vi "I2C Grove 8x8Matrix LED.vi"() -> ()   [LabVIEW 2020, in "CTI-Scratchpad.lvlib"]
uses:
  CTI-Scratchpad.lvlib
  CTI/Identity.ctl
  CTI-Peripheral/I2CLEDMatrix/Base/Data Types/ICONS.ctl
  CTI/Error Reporting.ctl
  CTI/I2C Address.ctl
  CTI/GPIO Number.ctl
  CTI/I2C Number.ctl
  CTI/Session/Session.lvclass
  CTI-Peripheral/I2CLEDMatrix/Grove I2C 8x8LEDMatrix/Grove I2C Matrix LED Driver.lvclass
  CTI/VisaComms/VisaComms.lvclass
  CTI/CTI.lvlib
  CTI-Peripheral/I2CLEDMatrix/Base/LEDMatrix.lvclass
panel:
  out "Shifting ASCII":bool[][](array[boolean])
  in  "Char":bool[][](array[boolean])=[[FALSE, FALSE, FALSE, FALSE, FALSE], [FALSE, FALSE, FALSE, FALSE, FALSE], [FALSE, FALSE, FALSE, FALSE, FALSE], [FALSE, FALSE, FALSE, FALSE, FALSE], [FALSE, FALSE, FALSE, FALSE, FALSE], [FALSE, FALSE, FALSE, FALSE, FALSE], [FALSE, FALSE, FALSE, FALSE, FALSE], [FALSE, FALSE, FALSE, FALSE, FALSE]]
  in  "Set Custom Char":bool
  in  "Set Scrolling Text":bool
  in  "Scrolling Text":string="test"
  in  "Icon":T1
  in  "Set Icon":bool
  in  "String":string
  in  "Set Char":bool
  out "Identity":T2
  in  "stop":bool
  in  "Grove Connector":enum16{"I2C0", "I2C1"}(ring)
  out "error out":errorcluster
  in  "Port":refnum<visa-resource-name>="COM4"
  # "https://wiki.seeedstudio.com/Grove-LED_Matrix_Driver-HT16K33/"
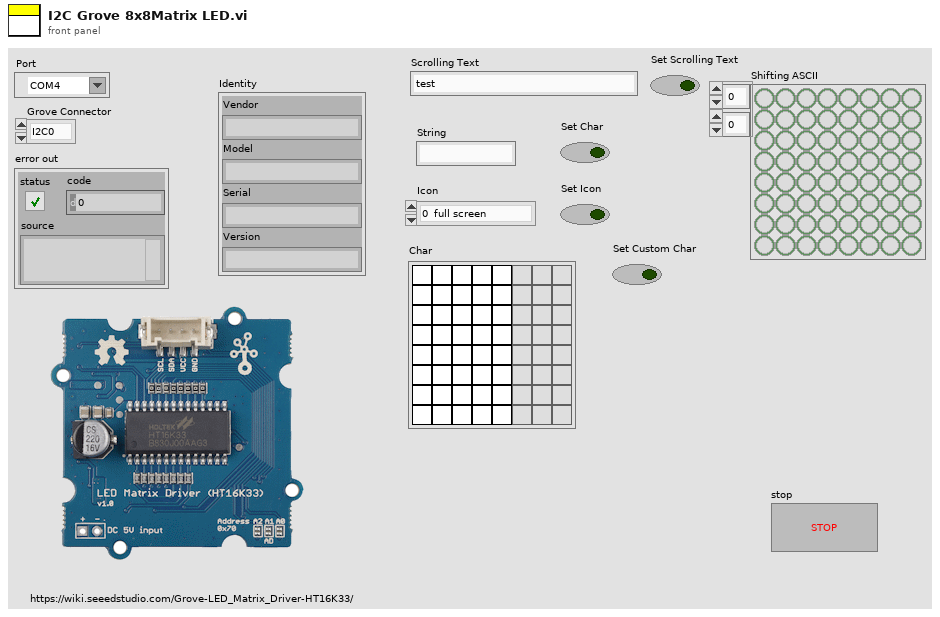
[diagram p1: front panel]
types:
  T1 = typedef "CTI-Peripheral.lvlib/LEDMatrix.lvclass/ICONS.ctl" = enum16{"0  full screen", "1  arrow_up", "2  arrow_down", "3  arrow_right", "4  arrow_left", "5  triangle_up", "6  triangle_down", "7  triangle_right", "8  triangel_left", "9  smile_face_1", "10 smile_face_2", "11 hearts", "12 diamonds", "13 clubs", "14 spades", "15 circle1", "16 circle2", "17 circle3", "18 circle4", "19 man", "20 woman", "21 musical_note_1", "22 musical_note_2", "23 snow", "24 up_down", "25 double_!", "26 left_right", "27 house"}
  T2 = typedef "CTI.lvlib/Identity.ctl" = cluster{"Vendor":string, "Model":string, "Serial":string, "Version":string}
  T3 = typedef "CTI.lvlib/I2C Address.ctl" = u8
  T4 = typedef "CTI.lvlib/Error Reporting.ctl" = enum16{"Minimal", "Moderate", "Full"}
  T5 = typedef "CTI.lvlib/I2C Number.ctl" = i8
  T6 = typedef "CTI.lvlib/GPIO Number.ctl" = i8
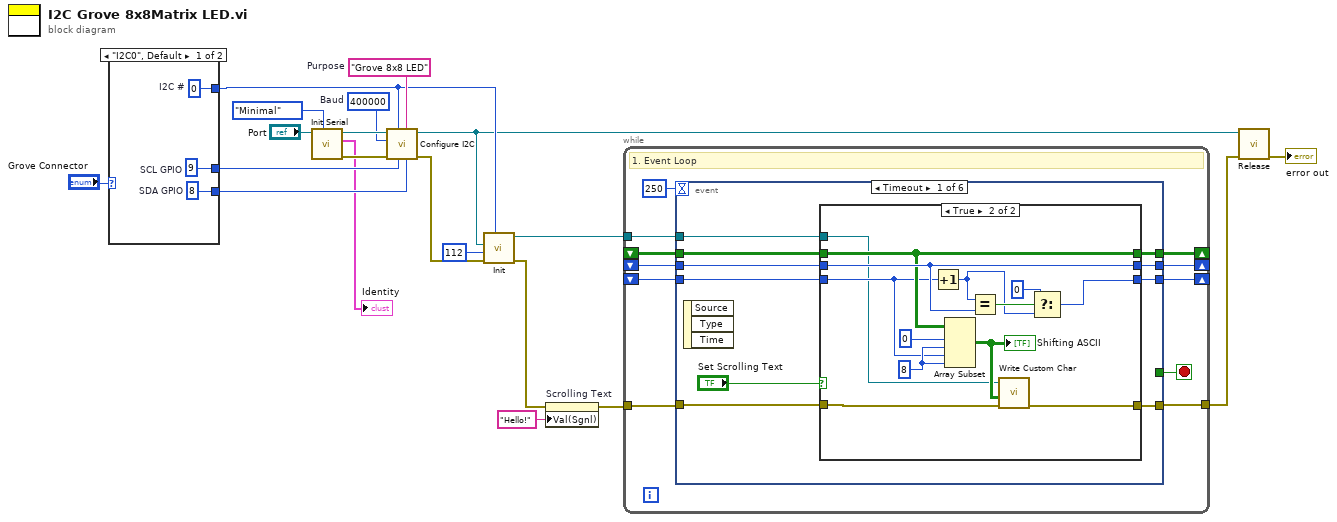
[diagram p0: block diagram]
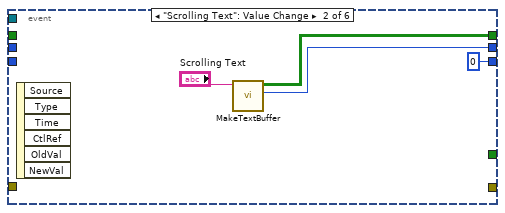
[diagram p3: hidden frame]
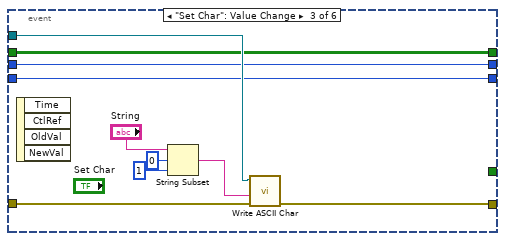
[diagram p4: hidden frame]
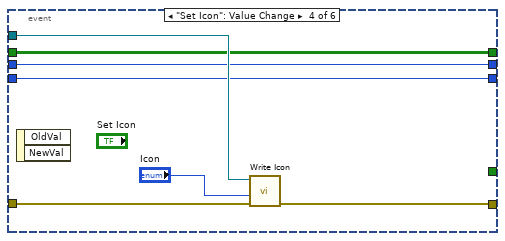
[diagram p5: hidden frame]
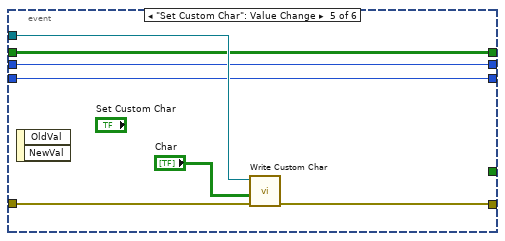
[diagram p6: hidden frame]
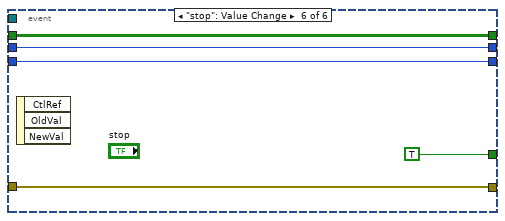
[diagram p7: hidden frame]
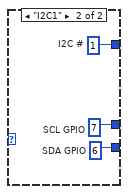
[diagram p8: hidden frame]
diagram:
  w15 = "Grove 8x8 LED"  # Purpose
  w16 = u32 400000  # Baud
  n1 = case shown="\"I2C0\", Default" "Grove Connector" {
    tunnel: [w23 w26] -> w13
    tunnel: [w22 w25] -> w12
    tunnel: [w21 w24] -> w8
    frame "I2C0", Default {
      w21 = T5 0  # I2C #
      w22 = T6 8  # SDA GPIO
      w23 = T6 9  # SCL GPIO
    }
    frame "I2C1" {
      w24 = T5 1  # I2C #
      w25 = T6 6  # SDA GPIO
      w26 = T6 7  # SCL GPIO
    }
  }
  n2 = call "Init Serial.vi"("Error Checking (Full)"=Error_Reporting."Minimal", "VISA resource name in"="Port") -> ("error out"=w17:errorcluster, "Identity"=→"Identity":T2, "Session"=w18:refnum<class "Session.lvclass">)  [unwired: 7 in]
  n3 = call "Configure I2C.vi"("SDA GPIO"=w12, "Purpose (\"I2C\")"=w15, "SCL GPIO"=w13, "I2C #"=w8, "error in (no error)"=w17, "Baud"=w16, "Session in"=w18) -> ("error out"=w5:errorcluster, "Session out"=w7:refnum<class "Session.lvclass">)  [unwired: 3 in]
  n4 = call "Init.vi"("I2C #"=w8, "error in (no error)"=w5, "Address"=T3 112, "Session In"=w7) -> ("error out"=w3:errorcluster, "Grove I2C Matrix LED Driver Out"=w4:refnum<class "Grove I2C Matrix LED Driver.lvclass">)  [unwired: 6 in]
  n5 = property on="Scrolling Text" class="Str"(error in=w3, "Val(Sgnl)"="Hello!" ("Value (Signaling)")) -> (error out=w2:errorcluster)  [unwired: 1 in, 1 out]
  n6 = while {
    tunnel: w2 -> [w36]
    tunnel: [w35] -> w10
    tunnel: w4 -> [w37]
    shift-right: [w32] -> _
    shift-left: _ -> [w31]
    shift-right: [w30] -> _
    shift-left: _ -> [w29]
    shift-right: [w27] -> _
    shift-left: _ -> [w28]
    stop <- w34 stop-if-true
    # "1. Event Loop"
    n7 = event shown="[0] Timeout" {
      selector: _ -> [_ _ _ _ _ _]
      dyn-events: _ -> [_ _ _ _ _ _]
      timeout: 250 -> [_ _ _ _ _ _]
      tunnel: w37 -> [w41 _ w76 w82 w90 _]
      tunnel: w36 -> [w40 _ w78 w85 w92 w97]
      tunnel: [w39 _ w77 w84 w91 w97] -> w35
      tunnel: [_ _ _ _ _ TRUE] -> w34
      tunnel: [w43 w67 w69 w81 w86 w93] -> w32
      tunnel: w31 -> [w44 _ w69 w81 w86 w93]
      tunnel: [w42 w66 w70 w79 w87 w94] -> w30
      tunnel: w29 -> [w45 _ w70 w79 w87 w94]
      tunnel: w28 -> [w47 _ w71 w80 w88 w95]
      tunnel: [w46 0 ("index") w71 w80 w88 w95] -> w27
      event Timeout {
        n8 = event-data() -> ()  [unwired: 1 in, 3 out]
        n9 = case shown="True" "Set Scrolling Text" {
          tunnel: w47 -> [w48 w56]
          tunnel: [w48 w62] -> w46
          tunnel: w45 -> [w49 w60]
          tunnel: w44 -> [w50 w57]
          tunnel: [w50 w57] -> w43
          tunnel: [w49 w60] -> w42
          tunnel: w41 -> [_ w52]
          tunnel: w40 -> [w51 w55]
          tunnel: [w51 w53] -> w39
          frame False {
          }
          frame True {
            w58 = 8 ("length")
            n10 = Increment(x=w56) -> (x+1=w61:i32)
            n11 = Array Subset(array=w57, index (row)=0 ("index"), length (row)=w58, index (col)=w56, length (col)=w58) -> (w54:bool[][])
            "Shifting ASCII" <- w54
            n12 = Equal?(x=w61, y=w60) -> (x = y?=w63:bool)
            n13 = call-dynamic "Write Custom Char.vi"("error in (no error)"=w55, "Char"=w54, "Grove I2C Matrix LED in"=w52) -> ("error out"=w53:errorcluster)  [unwired: 7 in, 1 out]
            n14 = Select(t=0 ("index"), s=w63, f=w61) -> (s? t:f=w62:i32)
          }
        }
      }
      event "Scrolling Text": Value Change {
        n15 = event-data() -> ()  [unwired: 1 in, 6 out]
        n16 = call "MakeTextBuffer.vi"("Text"="Scrolling Text") -> ("size"=w66:i32, "Buffer"=w67:bool[][])  [unwired: 9 in]
      }
      event "Set Char": Value Change {
        n17 = event-data() -> ()  [unwired: 1 in, 4 out]
        n18 = String Subset(string="String", offset (0)=0, length (rest)=1 ("length (rest)")) -> (substring=w72:string)
        n19 = call-dynamic "Write ASCII Char.vi"("error in (no error)"=w78, "Char"=w72, "Grove I2C Matrix LED Driver in"=w76) -> ("error out"=w77:errorcluster)  [unwired: 7 in, 1 out]
      }
      event "Set Icon": Value Change {
        n20 = event-data() -> ()  [unwired: 1 in, 2 out]
        n21 = call-dynamic "Write Icon.vi"("error in (no error)"=w85, "Icon"="Icon", "Grove I2C Matrix LED in"=w82) -> ("error out"=w84:errorcluster)  [unwired: 7 in, 1 out]
      }
      event "Set Custom Char": Value Change {
        n22 = event-data() -> ()  [unwired: 1 in, 2 out]
        n23 = call-dynamic "Write Custom Char.vi"("error in (no error)"=w92, "Char"="Char", "Grove I2C Matrix LED in"=w90) -> ("error out"=w91:errorcluster)  [unwired: 7 in, 1 out]
      }
      event "stop": Value Change {
        n24 = event-data() -> ()  [unwired: 1 in, 3 out]
      }
    }
  }
  n25 = call-dynamic "Release.vi"("error in (no error)"=w10, "Session in"=w7) -> ("error out"=→"error out":errorcluster)  [unwired: 9 in]
